vi "SVL Set dB Reference (N Ch - 1 Ref).vi"(8 "error in (no error)":errorcluster, 10 "dB reference [EU]":dbl=1.0 format="%^.1e", 11 "scaled signals in [EU]":waveform(dbl)[](array[waveform])=[{"t0"=timestamp(0 s since 1904-01-01), "dt"=0.0, "Y"=[]}]) -> (0 "error out":errorcluster, 3 "scaled signals out [EU]":waveform(dbl)[](array[waveform]))   [LabVIEW 2017]
doc: "Sets the specified <B>dB reference [EU]</B> as an attribute in the <B>scaled signal out [EU]</B> waveform. <B>dB reference [EU]</B> is used for all downstream conversions to dB. Wire data to the <B>scaled signal in [EU]</B> input to determine the polymorphic instance to use or manually select the instance."
uses:
  <vilib>/addons/_NISVFA/_Shared subVIs/Common/SVL Set dB Reference (variant).vi
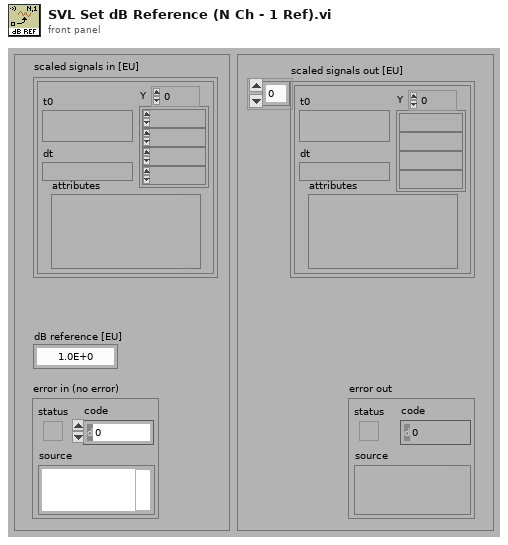
[diagram p1: front panel]
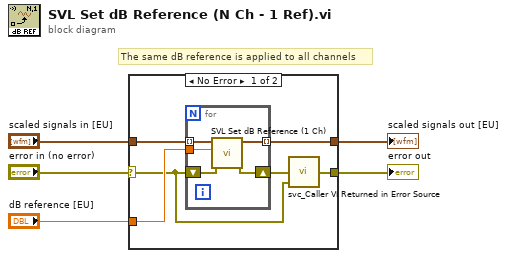
[diagram p0: block diagram]
diagram:
  # "The same dB reference is applied to all channels"
  n1 = case shown="No Error" "error in (no error)" {
    selector: "error in (no error)" -> [w6 w18]
    tunnel: "scaled signals in [EU]" -> [w10 w17]
    tunnel: [w11 w18] -> w4
    tunnel: [w9 w17] -> w3
    tunnel: "dB reference [EU]" -> [w8 _]
    frame No Error {
      n2 = for {
        tunnel: w10 -> [w16] mode=indexing
        tunnel: [w15] -> w9 mode=indexing
        tunnel: w8 -> [w14]
        shift-right: [w13] -> w7
        shift-left: w6 -> [w12]
        n3 = call <vilib>:"SVL Set dB Reference (1 Ch).vi"("error in (no error)"=w12, "dB reference [EU]"=w14, "scaled signal in [EU]"=w16) -> ("error out"=w13:errorcluster, "scaled signal out [EU]"=w15:waveform(dbl))  [unwired: 7 in]
      }
      n4 = call <vilib>:"svc_Caller VI Returned in Error Source.vi"("warning input to caller"=w6, "error in (no error)"=w7) -> ("error out"=w11:errorcluster)  [unwired: 3 in]
    }
    frame Error {
    }
  }
  "scaled signals out [EU]" <- w3
  "error out" <- w4
